vi "KE2260B Display Text.vi"(6 "Display Text":string, 8 "error in (no error)":errorcluster, 9 "Display Blink (F : disable)":bool, 10 "Clear Text (F : disable)":bool, 11 "VISA resource name":refnum<visa-resource-name>) -> (0 "error out":errorcluster, 3 "VISA resource name out":refnum<visa-resource-name>)   [LabVIEW 2009, in "Keithley 2260B.lvlib"]
doc: "Display text and blinking."
uses:
  <instrlib>/Keithley 2260B/Keithley 2260B.lvlib
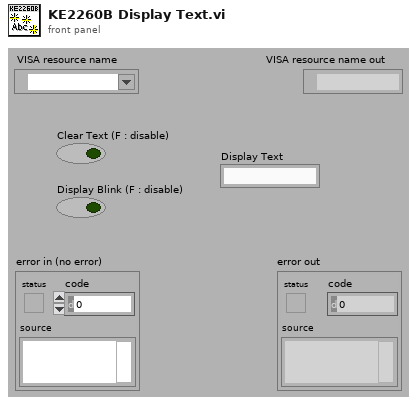
[diagram p1: front panel]
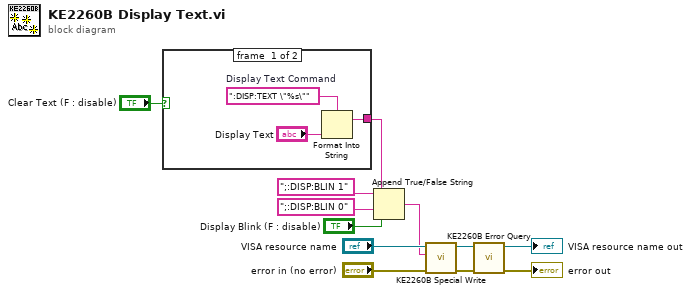
[diagram p0: block diagram]
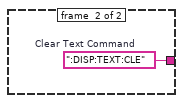
[diagram p2: hidden frame]
diagram:
  n1 = case shown="False" "Clear Text (F : disable)" {
    tunnel: [w14 w16] -> w5
    frame #0 {
      w15 = ":DISP:TEXT \"%s\""  # Display Text Command
      n2 = Format Into String(format string=w15, "Display Text") -> (resulting string=w14:string)  [unwired: 2 in, 1 out]
    }
    frame #1 {
      w16 = ":DISP:TEXT:CLE"  # Clear Text Command
    }
  }
  n3 = Append True/False String(1:"Display Blink (F : disable)", 2:";:DISP:BLIN 0" ("false string"), 3:";:DISP:BLIN 1" ("true string"), 4:w5) -> (0:w1:string)
  n4 = call <instrlib>:"KE2260B Special Write.vi"("error in (no error)"="error in (no error)", "Write Buffer (\"\")"=w1, "VISA session"="VISA resource name") -> ("error out"=w10:errorcluster, "dup VISA session"=w9:refnum<visa-resource-name>)  [unwired: 6 in, 1 out]
  n5 = call <instrlib>:"KE2260B Error Query.vi"("error in (no error)"=w10, "VISA resource name"=w9) -> ("error out"=→"error out":errorcluster, "VISA resource name out"=→"VISA resource name out":refnum<visa-resource-name>)  [unwired: 6 in, 2 out]
